vi "start_pulse_task.vi"(8 "error in":errorcluster, 11 "Clock In":refnum<class "ClockDL100201DAQmx.lvclass">) -> (0 "error out":errorcluster, 3 "Clock Out":refnum<class "ClockDL100201DAQmx.lvclass">)   [LabVIEW 2010, in "ClockDL100201DAQmx.lvclass"]
uses:
  ClockDL100201DAQmx.lvclass
  ClockDL100201DAQmx.lvclass/ClockDL100201DAQmx.ctl
  <vilib>/DAQmx/write.llb/DAQmx Write (Digital 1D U8 1Chan NSamp).vi
  <vilib>/DAQmx/create/channels.llb/DAQmx Create Channel (DO-Digital Output).vi
  <vilib>/DAQmx/configure/timing.llb/DAQmx Timing (Sample Clock).vi
  <vilib>/DAQmx/configure/trigger.llb/DAQmx Start Trigger (Digital Edge).vi
  <vilib>/daqmx/miscellaneous.llb/DAQmx Fill In Error Info.vi
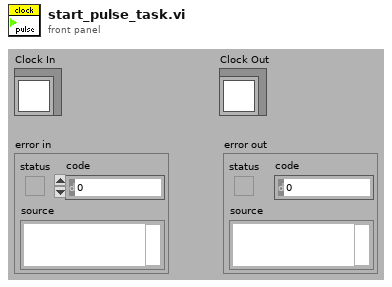
[diagram p1: front panel]
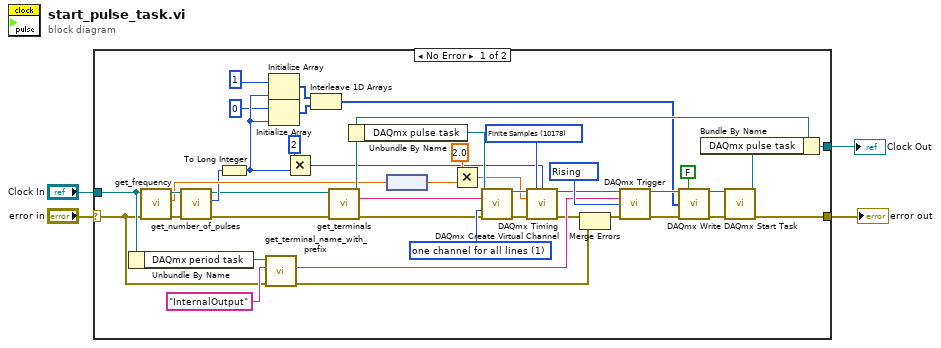
[diagram p0: block diagram]
diagram:
  n1 = case shown="No Error" "error in" {
    selector: "error in" -> [w30 w48]
    tunnel: "Clock In" -> [w42 w49]
    tunnel: [w40 w48] -> w3
    tunnel: [w39 w49] -> w2
    frame No Error {
      w29 = 1 items=["one channel for each line", "one channel for all lines"] ("line grouping")
      w47 = 10280 items=["Rising"=10280, "Falling"=10171] ("edge")
      w32 = 10178 items=["Finite Samples"=10178, "Continuous Samples"=10123, "Hardware Timed Single Point"=12522] ("sample mode")
      n2 = Unbundle By Name(w42) -> ("DAQmx period task"=w43:refnum<k21>)
      n3 = call-dynamic "get_frequency.vi"("error in (no error)"=w30, "GenericClock.lvclass in"=w42) -> ("error out"=w36:errorcluster, "frequency"=w28:dbl[unit], "GenericClock.lvclass out"=w37:refnum<class "ClockDL100201DAQmx.lvclass">)  [unwired: 7 in]
      n4 = call-dynamic "get_number_of_pulses.vi"("error in (no error)"=w36, "GenericClock.lvclass in"=w37) -> ("error out"=w9:errorcluster, "number of pulses"=w23:i64, "GenericClock.lvclass out"=w10:refnum<class "ClockDL100201DAQmx.lvclass">)  [unwired: 7 in]
      n5 = To Long Integer(number=w23) -> (32bit integer=w21:i32)
      n6 = call "get_terminal_name_with_prefix.vi"("error in (no error)"=w30, "Local Terminal Name"="InternalOutput", "task in"=w43) -> ("error out"=w45:errorcluster, "Terminal Name with Device Prefix"=w46:tag)  [unwired: 6 in, 1 out]
      n7 = Initialize Array(u8 1, w21) -> (w18:u8[])
      n8 = Initialize Array(u8 0, w21) -> (w17:u8[])
      n9 = Multiply(x=2, y=w21) -> (x*y=w22:i32)
      n10 = Interleave 1D Arrays(w18, w17) -> (w11:u8[])
      n11 = call-dynamic "get_terminals.vi"("ClockDL100201DAQmx in"=w10, "error in (no error)"=w9) -> ("ClockDL100201DAQmx out"=w38:refnum<class "ClockDL100201DAQmx.lvclass">, "output terminal"=w8:tag, "error out"=w7:errorcluster)  [unwired: 9 in, 2 out]
      n12 = Unbundle By Name(w38) -> ("DAQmx pulse task"=w41:refnum<k21>)
      n13 = node(w28) -> (w26:dbl)
      n14 = Multiply(x=2.0 ("y"), y=w26) -> (x*y=w27:dbl)
      n15 = call-poly <vilib>:"DAQmx Create Virtual Channel.vi"("task in"=w41, "lines"=w8, "line grouping"=w29, "error in"=w7) -> ("task out"=w33:refnum<k21>, "error out"=w34:errorcluster)  [unwired: 10 in]
      n16 = call-poly <vilib>:"DAQmx Timing.vi"("task/channels in"=w33, "sample mode"=w32, "samples per channel"=w22, "rate"=w27, "error in"=w34) -> ("task out"=w35:refnum<k21>, "error out"=w6:errorcluster)  [unwired: 9 in]
      n17 = Merge Errors(w6, w45) -> (w5:errorcluster)
      n18 = call-poly <vilib>:"DAQmx Trigger.vi"("task/channels in"=w35, "source"=w46, "edge"=w47, "error in"=w5) -> ("task out"=w16:refnum<k21>, "error out"=w15:errorcluster)  [unwired: 10 in]
      n19 = call-poly <vilib>:"DAQmx Write.vi"("task/channels in"=w16, "auto start"=FALSE, "data"=w11, "error in"=w15) -> ("task out"=w14:refnum<k21>, "error out"=w13:errorcluster)  [unwired: 9 in, 1 out]
      n20 = call <vilib>:"DAQmx Start Task.vi"("task/channels in"=w14, "error in"=w13) -> ("task out"=w31:refnum<k21>, "error out"=w40:errorcluster)  [unwired: 12 in]
      n21 = Bundle By Name(cluster=w38, "DAQmx pulse task"=w31) -> (w39:refnum<class "ClockDL100201DAQmx.lvclass">)
    }
    frame Error {
    }
  }
  "error out" <- w3
  "Clock Out" <- w2
